vi "Configure Acquisition.vi"(8 "error in":errorcluster, 11 "IMAQdx Triggered Continuous Acquisition in":refnum<class "IMAQdx Triggered Continuous Acquisition.lvclass">) -> (0 "error out":errorcluster, 3 "IMAQdx Triggered Continuous Acquisition out":refnum<class "IMAQdx Triggered Continuous Acquisition.lvclass">)   [LabVIEW 2024, in "IMAQdx Triggered Continuous Acquisition.lvclass"]
uses:
  IMAQdx Triggered Continuous Acquisition.lvclass
  IMAQdx Triggered Continuous Acquisition.lvclass/IMAQdx Triggered Continuous Acquisition.ctl
  Base/IMAQdx Base Configure Strategy.lvclass
  <vilib>/vision/driver/NI_Vision_Acquisition_Software.lvlib
  <vilib>/vision/driver/IMAQdx.llb/IMAQdx Acquisition Mode.ctl
  Source/Interfaces/IConfiguration/IConfiguration.lvclass
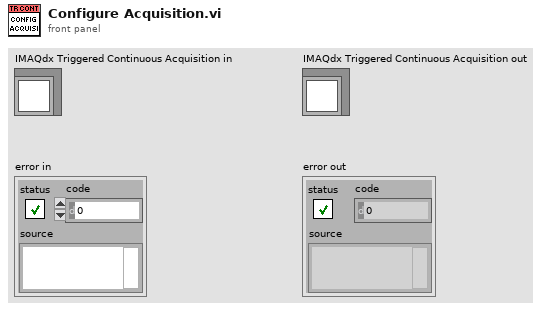
[diagram p1: front panel]
types:
  T1 = typedef "NI_Vision_Acquisition_Software.lvlib/IMAQdx Acquisition Mode.ctl" = enum32{"One Shot", "Continuous"}
  T2 = typedef "Generic Image.lvclass/Pixel Format.ctl" = enum16{"Grayscale (U8)", "Grayscale (I16)", "Grayscale (SGL)", "Complex (CSG)", "RGB (U32)", "HSL (U32)", "RGB (U64)", "Grayscale (U16)"}
  T3 = typedef "Image Type" = u32
  T4 = typedef "IMAQ Image.ctl" = refnum<image>
  T5 = typedef "IMAQdx.ctl" = refnum<k21>
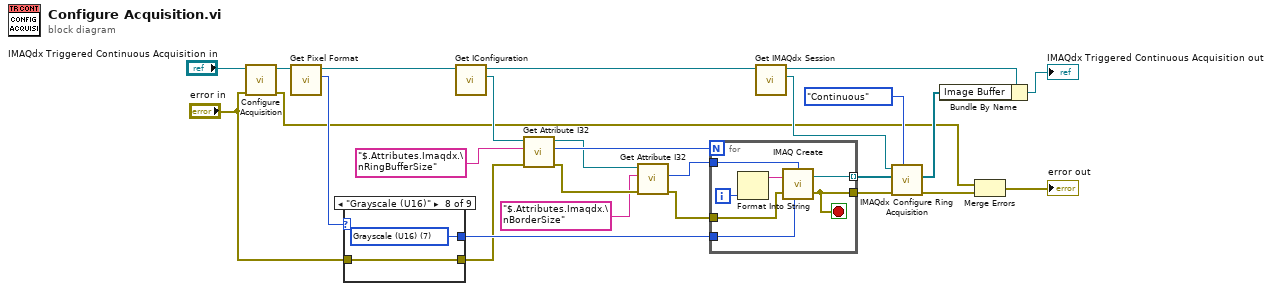
[diagram p0: block diagram]
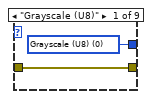
[diagram p2: hidden frame]
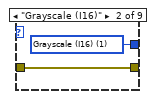
[diagram p3: hidden frame]
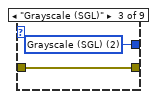
[diagram p4: hidden frame]
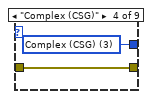
[diagram p5: hidden frame]
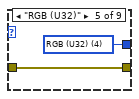
[diagram p6: hidden frame]
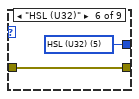
[diagram p7: hidden frame]
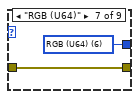
[diagram p8: hidden frame]
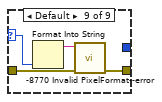
[diagram p9: hidden frame]
diagram:
  n1 = call-parent "Configure Acquisition.vi"("error in"="error in", "IMAQdx Base Configure Strategy in"="IMAQdx Triggered Continuous Acquisition in") -> ("error out"=w1:errorcluster, "IMAQdx Base Configure Strategy out"=w23:refnum<class "IMAQdx Triggered Continuous Acquisition.lvclass">)  [unwired: 8 in]
  n2 = call "Get Pixel Format.vi"("IMAQdx Base Configure Strategy in"=w23) -> ("Pixel Format"=w12:T2, "IMAQdx Base Configure Strategy out"=w13:refnum<class "IMAQdx Triggered Continuous Acquisition.lvclass">)  [unwired: 9 in]
  n3 = case shown="\"Grayscale (U16)\"" w12 {
    selector: w12 -> [_ _ _ _ _ _ _ _ w43]
    tunnel: [w28 w30 w32 w34 w36 w38 w40 w42 _] -> w11
    tunnel: "error in" -> [w27 w29 w31 w33 w35 w37 w39 w41 w46]
    tunnel: [w27 w29 w31 w33 w35 w37 w39 w41 w45] -> w10
    frame "Grayscale (U8)" {
      w28 = T3 0 items=["Grayscale (U8)", "Grayscale (I16)", "Grayscale (SGL)", "Complex (CSG)", "RGB (U32)", "HSL (U32)", "RGB (U64)", "Grayscale (U16)"] ("Image Type")
    }
    frame "Grayscale (I16)" {
      w30 = T3 1 items=["Grayscale (U8)", "Grayscale (I16)", "Grayscale (SGL)", "Complex (CSG)", "RGB (U32)", "HSL (U32)", "RGB (U64)", "Grayscale (U16)"] ("Image Type")
    }
    frame "Grayscale (SGL)" {
      w32 = T3 2 items=["Grayscale (U8)", "Grayscale (I16)", "Grayscale (SGL)", "Complex (CSG)", "RGB (U32)", "HSL (U32)", "RGB (U64)", "Grayscale (U16)"] ("Image Type")
    }
    frame "Complex (CSG)" {
      w34 = T3 3 items=["Grayscale (U8)", "Grayscale (I16)", "Grayscale (SGL)", "Complex (CSG)", "RGB (U32)", "HSL (U32)", "RGB (U64)", "Grayscale (U16)"] ("Image Type")
    }
    frame "RGB (U32)" {
      w36 = T3 4 items=["Grayscale (U8)", "Grayscale (I16)", "Grayscale (SGL)", "Complex (CSG)", "RGB (U32)", "HSL (U32)", "RGB (U64)", "Grayscale (U16)"] ("Image Type")
    }
    frame "HSL (U32)" {
      w38 = T3 5 items=["Grayscale (U8)", "Grayscale (I16)", "Grayscale (SGL)", "Complex (CSG)", "RGB (U32)", "HSL (U32)", "RGB (U64)", "Grayscale (U16)"] ("Image Type")
    }
    frame "RGB (U64)" {
      w40 = T3 6 items=["Grayscale (U8)", "Grayscale (I16)", "Grayscale (SGL)", "Complex (CSG)", "RGB (U32)", "HSL (U32)", "RGB (U64)", "Grayscale (U16)"] ("Image Type")
    }
    frame "Grayscale (U16)" {
      w42 = T3 7 items=["Grayscale (U8)", "Grayscale (I16)", "Grayscale (SGL)", "Complex (CSG)", "RGB (U32)", "HSL (U32)", "RGB (U64)", "Grayscale (U16)"] ("Image Type")
    }
    frame Default {
      n4 = Format Into String(w43) -> (resulting string=w44:string)  [unwired: 3 in, 1 out]
      n5 = call "-8770 Invalid PixelFormat--error.vi"("error in"=w46, "Argument"=w44) -> ("error out"=w45:errorcluster)  [unwired: 9 in]
    }
  }
  n6 = call-dynamic "Get IConfiguration.vi"("IMAQdx Base Configure Strategy in"=w13) -> ("IConfiguration"=w22:refnum<class "IConfiguration.lvclass">, "IMAQdx Base Configure Strategy out"=w9:refnum<class "IMAQdx Triggered Continuous Acquisition.lvclass">)  [unwired: 9 in]
  n7 = call-dynamic "Get Attribute I32.vi"("error in"=w10, "Attribute"="$.Attributes.Imaqdx.\nRingBufferSize", "IConfiguration in"=w22) -> ("error out"=w7:errorcluster, "Value"=w19:i32, "IConfiguration out"=w8:refnum<class "IConfiguration.lvclass">)  [unwired: 6 in]
  n8 = call-dynamic "Get Attribute I32.vi"("error in"=w7, "Attribute"="$.Attributes.Imaqdx.\nBorderSize", "IConfiguration in"=w8) -> ("error out"=w4:errorcluster, "Value"=w5:i32)  [unwired: 6 in, 1 out]
  n9 = for {
    N: w19 -> [_]
    tunnel: w4 -> [w51]
    tunnel: [w50] -> w18
    tunnel: [w49] -> w17 mode=indexing
    tunnel: w11 -> [w48]
    tunnel: w5 -> [w47]
    i -> [w53]
    stop <- w50 stop-if-true
    n10 = Format Into String(w53) -> (resulting string=w52:string)  [unwired: 3 in, 1 out]
    n11 = call "IMAQ Create"("Border Size"=w47, "Image Name"=w52, "Image Type"=w48, "error in (no error)"=w51) -> ("New Image"=w49:T4, "error out"=w50:errorcluster)  [unwired: 1 in]
  }
  n12 = call "Get IMAQdx Session.vi"("IMAQdx Base Configure Strategy in"=w9) -> ("IMAQdx Session"=w24:T5, "IMAQdx Base Configure Strategy out"=w25:refnum<class "IMAQdx Triggered Continuous Acquisition.lvclass">)  [unwired: 9 in]
  n13 = call <vilib>:"IMAQdx Configure Ring Acquisition.vi"("Mode"=IMAQdx_Acquisition_Mode."Continuous", "error in"=w18, "Images"=w17, "Session In"=w24) -> ("error out"=w16:errorcluster, "Images Out"=w14:T4[])  [unwired: 5 in, 1 out]
  n14 = Bundle By Name(cluster=w25, "Image Buffer"=w14) -> (→"IMAQdx Triggered Continuous Acquisition out":refnum<class "IMAQdx Triggered Continuous Acquisition.lvclass">)
  n15 = Merge Errors(w1, w16) -> (→"error out":errorcluster)
